vi "dfd_Validate NStage MRate Quantization.vi"(8 "error in (no error)":errorcluster, 10 "coef wl":i16[](array[numeric]), 11 "multirate filters in":T1[](array[typedef]) {"mMRate_SumWl" min=1 max=32 step=1; "mMRate_InputIwl" min=1 max=32 step=1; "mMRate_GainWl" min=1 max=32 step=1; "mMRate_OutputWl" min=1 max=32 step=1; "mMRate_InputWl" min=1 max=32 step=1; "mMRate_CoefWl" min=1 max=32 step=1; "mMRate_Mode" items=["Default"=-1, "No Rate Change"=0, "Interpolation"=1, "Decimation"=2, "Interpolated"=3, "Rational"=4]}) -> (0 "error out":errorcluster, 1 "last FIR idx":i32, 2 "dup coef wl":i16[](array[numeric]), 3 "dup multirate filters in":T1[](array[typedef]) {"mMRate_SumWl" min=1 max=32 step=1; "mMRate_InputIwl" min=1 max=32 step=1; "mMRate_GainWl" min=1 max=32 step=1; "mMRate_OutputWl" min=1 max=32 step=1; "mMRate_InputWl" min=1 max=32 step=1; "mMRate_CoefWl" min=1 max=32 step=1; "mMRate_Mode" items=["Default"=-1, "No Rate Change"=0, "Interpolation"=1, "Decimation"=2, "Interpolated"=3, "Rational"=4]})   [LabVIEW 2017, in "NI_DigFilter_FXP.lvlib"]
uses:
  <vilib>/addons/Digital Filter Design/NI_DigFilter_FXP.lvlib
  <vilib>/addons/Digital Filter Design/_Objects.llb/DFD Multirate Filter Obj.ctl
  <vilib>/addons/Digital Filter Design/_Objects.llb/DFD Multirate Mode.ctl
  <vilib>/addons/Digital Filter Design/_Objects.llb/DFD Coef Norm Type.ctl
  <vilib>/addons/Digital Filter Design/_Objects.llb/DFD Round-off Mode.ctl
  <vilib>/addons/Digital Filter Design/_Objects.llb/DFD FXP MRate Multiply Mode.ctl
  <vilib>/addons/Digital Filter Design/_Misc.llb/dfd_Error Handlers (Single).vi
  <vilib>/addons/Digital Filter Design/NI_DigFilterLicensed.lvlib
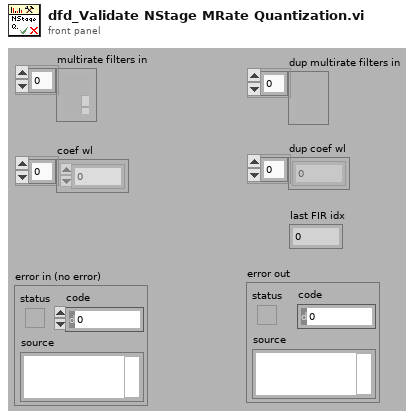
[diagram p1: front panel]
types:
  T1 = typedef "NI_DigFilterLicensed.lvlib/DFD Multirate Filter Obj.ctl" = cluster{"mMRate_Structure":enum16{"CIC", "FIR", "IIR", "Lattice"}, "mMRate_Mode":T2, "mMRate_Factor":i32, "mMRate_FIRParams":cluster{"mMRate_FIR_H":dbl[], "mMRate_FIR_IsNyquist?":bool, "mMRate_FIR_IsSymmetric?":bool}, "mMRate_CICParams":cluster{"mMRate_CIC_#Stage":i32, "mMRate_CIC_Lag":i32, "mMRate_CIC_Type":enum16{"Lowpass", "Highpass"}}, "mMRate_Order":i32, "mMRate_Version":string, "mMRate_Comments":string, "mMRate_RationalFactor":cluster{"mMRate_L":i32, "mMRate_M":i32}, "mMRate_Fs":dbl, "mMRate_Quantized?":bool, "mMRate_QFilterGain":dbl, "mMRate_CoefWl":i16, "mMRate_Scaling":cluster{"mMRate_ScaleByPowerOf2?":bool, "mMRate_ScaleType":T3}, "mMRate_InputWl":i16, "mMRate_OutputWl":i16, "mMRate_OutputMode":T4, "mMRate_MultMode":T5, "mMRate_BitPruning":bool, "mMRate_GainWl":i16, "mMRate_OutputFwl":i16, "mMRate_SumIwl":i16, "mMRate_InputIwl ":i16, "mMRate_SumWl":i16, "mMRate_CoefIwl":i16}
  T2 = typedef "NI_DigFilterLicensed.lvlib/DFD Multirate Mode.ctl" = i16
  T3 = typedef "NI_DigFilterLicensed.lvlib/DFD Coef Norm Type.ctl" = enum16{"No Norm", "Time Domain 1-Norm", "Time Domain 2-Norm", "Time Domain Inf-Norm"}
  T4 = typedef "NI_DigFilterLicensed.lvlib/DFD Round-off Mode.ctl" = enum16{"Nearest", "Truncation"}
  T5 = typedef "NI_DigFilterLicensed.lvlib/DFD FXP MRate Multiply Mode.ctl" = enum16{"Truncated", "Full"}
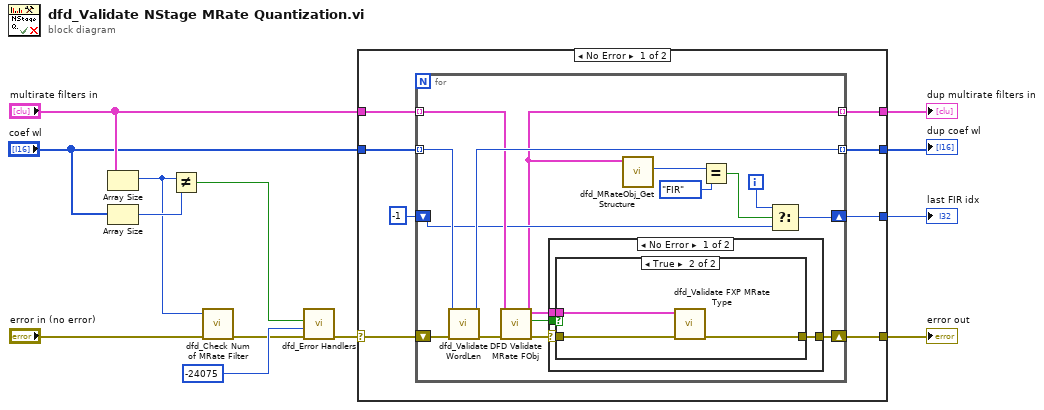
[diagram p0: block diagram]
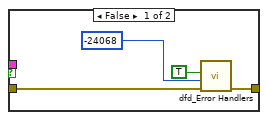
[diagram p2: hidden frame]
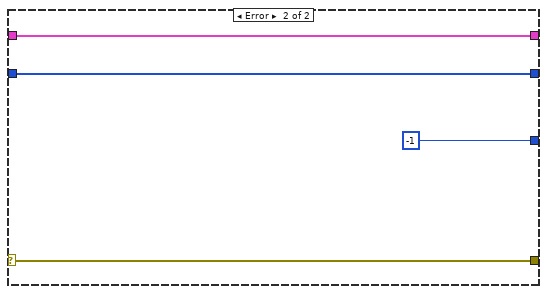
[diagram p4: hidden frame]
diagram:
  n1 = Array Size(array="multirate filters in") -> (size(s)=w8:i32)
  n2 = Array Size(array="coef wl") -> (size(s)=w11:i32)
  n3 = Not Equal?(x=w8, y=w11) -> (x != y?=w12:bool)
  n4 = call <vilib>:"dfd_Check Num of MRate Filter.vi"("error in (no error)"="error in (no error)", "#MRate in"=w8) -> ("error out"=w9:errorcluster)  [unwired: 9 out]
  n5 = call-poly <vilib>:"dfd_Error Handlers.vi"("error in (no error)"=w9, "error code"=-24075 ("ERR_COEF_WL_ARRAY_SIZE"), "condition failed?"=w12) -> ("error out"=w7:errorcluster)  [unwired: 8 out]
  n6 = case shown="No Error" w7 {
    selector: w7 -> [w21 w52]
    tunnel: "multirate filters in" -> [w20 w50]
    tunnel: "coef wl" -> [w19 w51]
    tunnel: [w16 w52] -> w1
    tunnel: [w18 w51] -> w3
    tunnel: [w17 w50] -> w2
    tunnel: [w14 -1] -> w4
    frame No Error {
      n7 = for {
        shift-right: [w30] -> w16
        shift-left: w21 -> [w36]
        tunnel: w20 -> [w32] mode=indexing
        tunnel: w19 -> [w35] mode=indexing
        tunnel: [w34] -> w18 mode=indexing
        tunnel: [w23] -> w17 mode=indexing
        shift-right: [w24] -> w14
        shift-left: -1 -> [w25]
        i -> [w26]
        n8 = call <vilib>:"dfd_Validate WordLen.vi"("error in (no error)"=w36, "wl"=w35) -> ("error out"=w33:errorcluster, "dup wl"=w34:i16)  [unwired: 8 out]
        n9 = call <vilib>:"DFD Validate MRate FObj.vi"("error in (no error)"=w33, "multirate filter in"=w32) -> ("error out"=w22:errorcluster, "is valid FLP?"=w31:bool, "multirate filter out"=w23:T1)  [unwired: 7 out]
        n10 = case shown="No Error" w22 {
          selector: w22 -> [w37 w48]
          tunnel: w31 -> [w40 _]
          tunnel: [w39 w48] -> w30
          tunnel: w23 -> [w38 _]
          frame No Error {
            n11 = case shown="True" w40 {
              tunnel: w37 -> [w44 w47]
              tunnel: [w43 w45] -> w39
              tunnel: w38 -> [_ w46]
              frame False {
                n12 = call-poly <vilib>:"dfd_Error Handlers.vi"("error in (no error)"=w44, "error code"=-24068 ("ERR_INVALID_FXP_MRATE"), "condition failed?"=TRUE) -> ("error out"=w43:errorcluster)  [unwired: 8 out]
              }
              frame True {
                n13 = call <vilib>:"dfd_Validate FXP MRate Type.vi"("error in (no error)"=w47, "multirate filter in"=w46) -> ("error out"=w45:errorcluster)  [unwired: 9 out]
              }
            }
          }
          frame Error {
          }
        }
        n14 = call <vilib>:"dfd_MRateObj_Get Structure.vi"("multirate filter in"=w23) -> ("structure"=w29:enum16{"CIC", "FIR", "IIR", "Lattice"})  [unwired: 10 out]
        n15 = Equal?(x=w29, y=enum16{"CIC", "FIR", "IIR", "Lattice"}."FIR") -> (x = y?=w27:bool)
        n16 = Select(t=w26, s=w27, f=w25) -> (s? t:f=w24:i32)
      }
    }
    frame Error {
    }
  }
  "error out" <- w1
  "dup multirate filters in" <- w2
  "dup coef wl" <- w3
  "last FIR idx" <- w4
